vi "EnetString.vi"(8 "error in (no error)":errorcluster, 9 "String":string, 10 "connection ID":refnum<k5>) -> (0 "error out":errorcluster, 1 "String out":string, 2 "connection ID 2":refnum<k5>)   [LabVIEW 2011]
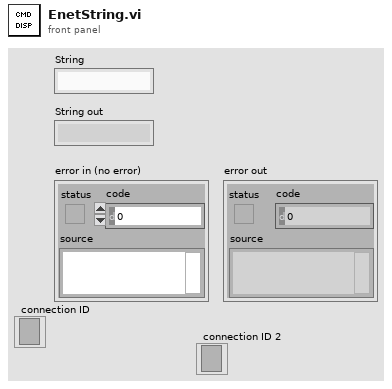
[diagram p1: front panel]
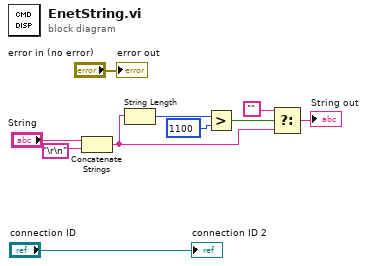
[diagram p0: block diagram]
diagram:
  n1 = Concatenate Strings("String", "\r\n") -> (w7:string)
  n2 = String Length(string=w7) -> (length=w5:i32)
  n3 = Greater?(x=w5, y=1100) -> (0:w3:bool)
  n4 = Select(t="", s=w3, f=w7) -> (s? t:f=→"String out":string)
  "error out" <- "error in (no error)"
  "connection ID 2" <- "connection ID"
